vi "Read Container Bounds Width.vi"(8 "error in (no error)":errorcluster, 11 "SubPanel.lvclass in":refnum<class "SubPanel.lvclass">) -> (0 "error out":errorcluster, 2 "Width":u32, 3 "SubPanel.lvclass out":refnum<class "SubPanel.lvclass">)   [LabVIEW 2015, in "SubPanel.lvclass"]
uses:
  SubPanel.lvclass
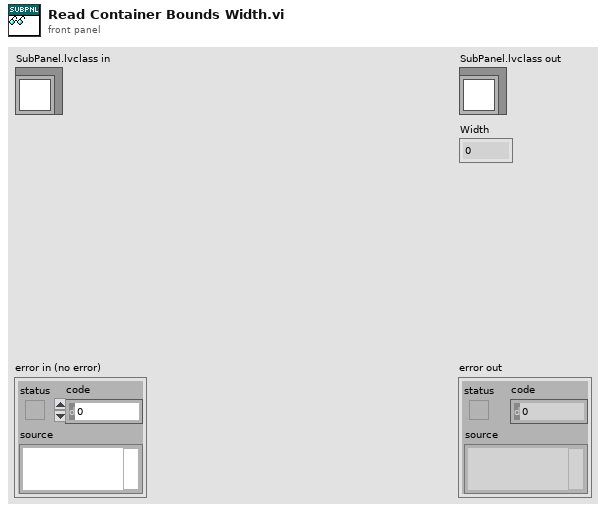
[diagram p1: front panel]
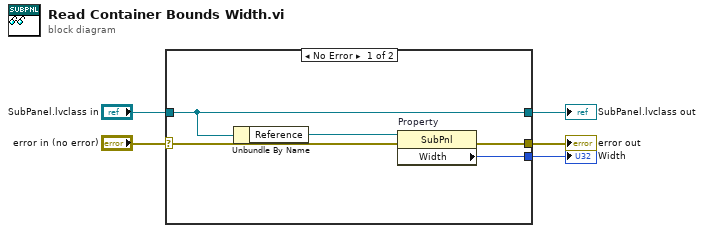
[diagram p0: block diagram]
diagram:
  n1 = case shown="No Error" "error in (no error)" {
    selector: "error in (no error)" -> [w6 w12]
    tunnel: [w9 w12] -> w4
    tunnel: [w8 w11] -> w2
    tunnel: "SubPanel.lvclass in" -> [w8 w11]
    tunnel: [w10 _] -> w1
    frame No Error {
      n2 = Unbundle By Name(w8) -> ("Reference"=w7:refnum<vi>)
      n3 = property on="Property" class="SubPnl"(reference=w7, error in=w6) -> (error out=w9:errorcluster, "Width"=w10:u32)  [unwired: 1 out]
    }
    frame Error {
    }
  }
  "error out" <- w4
  "SubPanel.lvclass out" <- w2
  "Width" <- w1
